vi "Configure Memory and Pressure.vi"(8 "error in (no error)":errorcluster, 9 "Memory Location (000)":i16 min=0 max=399 step=1 format="%0#3.0f", 10 "Pressure Setting (0000)":i16 min=0 max=1000 step=1 format="%04.0f", 11 "VISA resource name":refnum<visa-resource-name>) -> (0 "error out":errorcluster, 3 "VISA resource name out":refnum<visa-resource-name>)   [LabVIEW 2018, in "EFD Ultimus V.lvlib"]
doc: "Updates the pressure value in the memory location specified in the command. This command will update the LCD screen to the specified memory location.\n\nHost Format: PH--CHcccPpppp\n ccc: The 3 digit memory location from 0-399. \n pppp: The four digit pressure setting excluding the decimal point. This is a unit less value. The valid\n pressure ranges and decimal point are determined by the pressure units currently selected in\n the dispenser"
uses:
  EFD Ultimus V.lvlib
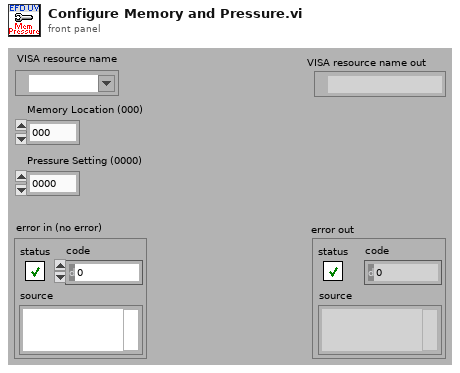
[diagram p1: front panel]
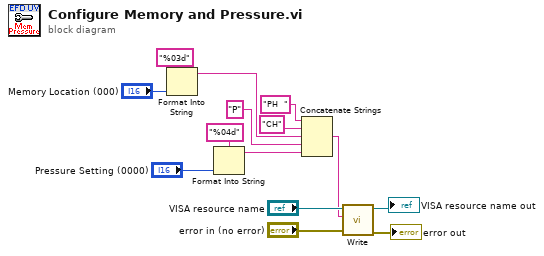
[diagram p0: block diagram]
diagram:
  n1 = Format Into String(format string="%03d", "Memory Location (000)") -> (resulting string=w4:string)  [unwired: 2 in, 1 out]
  n2 = Format Into String(format string="%04d", "Pressure Setting (0000)") -> (resulting string=w6:string)  [unwired: 2 in, 1 out]
  n3 = Concatenate Strings("PH  " ("string"), "CH" ("string"), w4, "P" ("string"), w6) -> (w9:string)
  n4 = call "Write.vi"("error in (no error)"="error in (no error)", "Command To Write"=w9, "VISA resource name"="VISA resource name") -> ("error out"=→"error out":errorcluster, "VISA resource name out"=→"VISA resource name out":refnum<visa-resource-name>)  [unwired: 7 out]
